vi "create new file.vi"(8 "error in":errorcluster, 10 "LogRotate in":refnum<class "LogRotate.lvclass">, 11 "logging path":path) -> (0 "error out":errorcluster, 3 "tdms file out":refnum<k34>)   [LabVIEW 2013, in "TDMS datalogger runtime.lvclass"]
uses:
  TDMS datalogger runtime.lvclass
  <vilib>/NI/LogRotate/LogRotate.lvclass
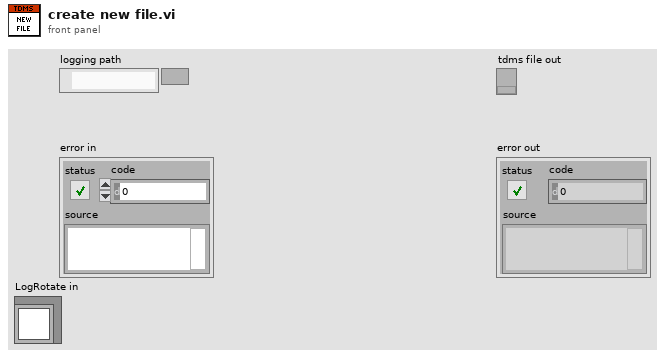
[diagram p1: front panel]
types:
  T1 = enum16{"open", "open or create", "create or replace", "create", "open (read-only)"}
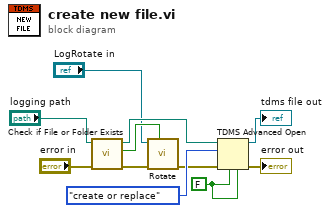
[diagram p0: block diagram]
diagram:
  w10 = FALSE ("disable buffering? (T)")
  n1 = call <vilib>:"Check if File or Folder Exists.vi"("error in (no error)"="error in", "path"="logging path") -> ("error out"=w7:errorcluster, "file or folder exists?"=w6:bool, "dup path"=w3:path)  [unwired: 7 in]
  n2 = call <vilib>:"Rotate.vi"("Force rotate"=w6, "error in (no error)"=w7, "LogRotate in"="LogRotate in") -> ("error out"=w2:errorcluster)  [unwired: 7 in, 1 out]
  n3 = TDMS Advanced Open(4:w10, 6:w10, 8:w2, 10:T1."create or replace" ("operation (0:open)"), 11:w3) -> (0:→"error out":errorcluster, 3:→"tdms file out":refnum<k34>)  [unwired: 1 out]
